vi "Write Persistence Path.vi"(8 "error in (no error)":errorcluster, 10 "Persistence Path":path, 11 "User Manager Model in":refnum<class "User Manager Model.lvclass">) -> (0 "error out":errorcluster, 3 "User Manager Model out":refnum<class "User Manager Model.lvclass">)   [LabVIEW 2017, in "User Manager Model.lvlib" / "User Manager Model.lvclass"]
uses:
  <vilib>/gpm_packages/@cs/User Manager App/User Manager Model/User Manager Model/User Manager Model.lvclass
  <vilib>/gpm_packages/@cs/User Manager App/User Manager Model/User Manager Model/User Manager Model.lvclass/User Manager Model.ctl
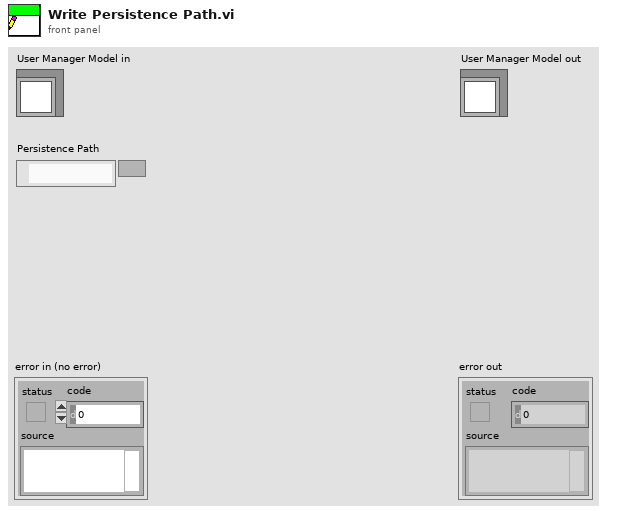
[diagram p1: front panel]
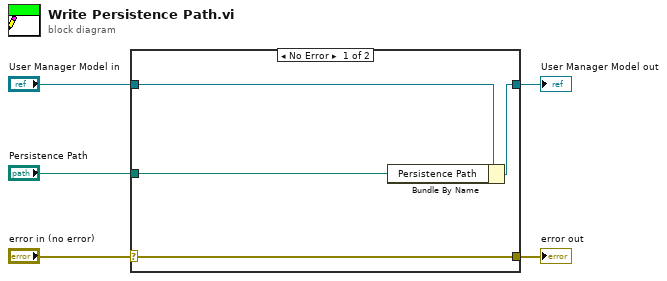
[diagram p0: block diagram]
diagram:
  n1 = case shown="No Error" "error in (no error)" {
    selector: "error in (no error)" -> [w9 w10]
    tunnel: [w9 w10] -> w4
    tunnel: [w7 w11] -> w2
    tunnel: "User Manager Model in" -> [w8 w11]
    tunnel: "Persistence Path" -> [w6 _]
    frame No Error {
      n2 = Bundle By Name(cluster=w8, "Persistence Path"=w6) -> (w7:refnum<class "User Manager Model.lvclass">)
    }
    frame Error {
    }
  }
  "error out" <- w4
  "User Manager Model out" <- w2
